vi "getDforce.vi"(6 "ForceDesired":dbl, 7 "Desired Direction":dbl[](array[numeric])) -> (3 "FX FY Fz 0 0 0":dbl[](array[numeric]))   [LabVIEW 2017]
uses:
  <vilib>/Analysis/_algsub.llb/Real Vector Norm.vi
  <vilib>/Analysis/NI_AALPro.lvlib
panel:
  out "norm F":dbl
  out "norm":dbl
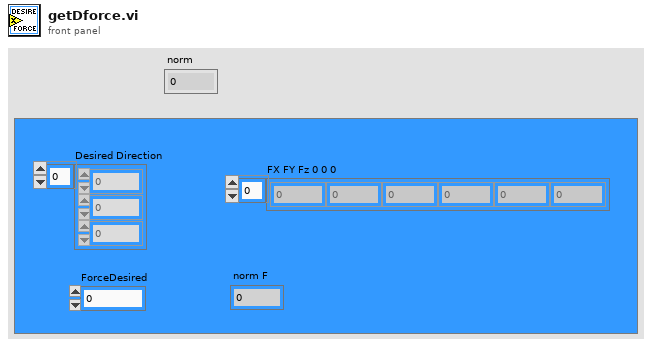
[diagram p1: front panel]
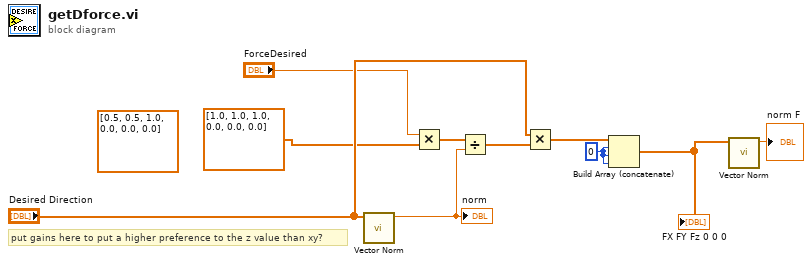
[diagram p0: block diagram]
diagram:
  (unwired) dbl[] [0.5, 0.5, 1.0, 0.0, 0.0, 0.0] ("DesiredFM_FF")
  w6 = 0
  # "put gains here to put a higher preference to the z value than xy?"
  n1 = call-poly <vilib>:"Vector Norm.vi"("Input Vector"="Desired Direction") -> ("norm"=w9:dbl)  [unwired: 9 in, 1 out]
  "norm" <- w9
  n2 = Multiply(x="ForceDesired", y=dbl[] [1.0, 1.0, 1.0, 0.0, 0.0, 0.0] ("DesiredFM_FF")) -> (x*y=w5:dbl[])
  n3 = Divide(x=w5, y=w9) -> (x/y=w10:dbl[])
  n4 = Multiply(x="Desired Direction", y=w10) -> (x*y=w7:dbl[])
  n5 = Build Array (concatenate)(w7, w6, w6, w6) -> (w3:dbl[])
  "FX FY Fz 0 0 0" <- w3
  n6 = call-poly <vilib>:"Vector Norm.vi"("Input Vector"=w3) -> ("norm"=→"norm F":dbl)  [unwired: 9 in, 1 out]
